vi "Build Coffee Shop.vi"(8 "error in (no error)":errorcluster) -> (0 "error out":errorcluster, 3 "Coffee Shop Out":refnum<class "Coffee Shop.lvclass">)   [LabVIEW 2020, in "Coffee Shop.lvclass"]
uses:
  Coffee Shop.lvclass
  Work Dispatcher/Work Dispatcher.lvclass
  C:/git/astemes-triarc-examples/source/Coffee Shop/Processes/People/Process Job/Job Handler.lvclass
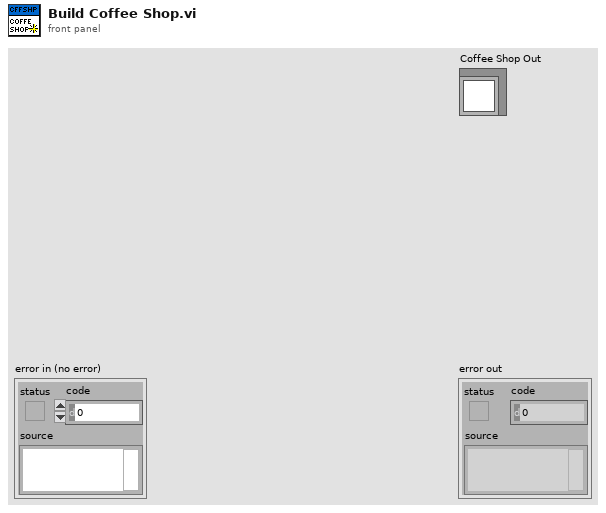
[diagram p1: front panel]
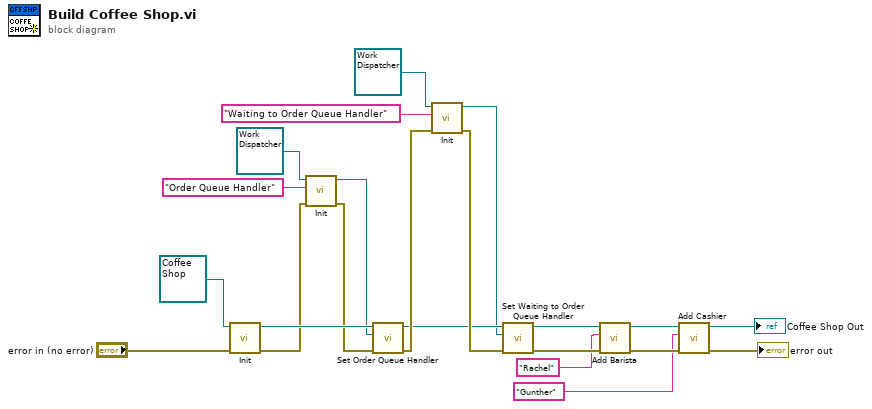
[diagram p0: block diagram]
diagram:
  n1 = call-dynamic "Init.vi"("error in (no error)"="error in (no error)", "Process In"=refnum<class "Coffee Shop.lvclass"> refnum ("Coffee Shop.lvclass")) -> ("error out"=w16:errorcluster, "Process Out"=w20:refnum<class "Coffee Shop.lvclass">)  [unwired: 8 in]
  n2 = call-dynamic "Init.vi"("error in (no error)"=w16, "Name"="Order Queue Handler", "Process In"=refnum<class "Work Dispatcher.lvclass"> refnum ("Work Dispatcher.lvclass")) -> ("error out"=w15:errorcluster, "Process Out"=w9:refnum<class "Work Dispatcher.lvclass">)  [unwired: 7 in]
  n3 = call "Set Order Queue Handler.vi"("error in (no error)"=w15, "Order Queue Handler"=w9, "Coffee Shop In"=w20) -> ("error out"=w13:errorcluster, "Coffee Shop Out"=w11:refnum<class "Coffee Shop.lvclass">)  [unwired: 7 in]
  n4 = call-dynamic "Init.vi"("error in (no error)"=w13, "Name"="Waiting to Order Queue Handler", "Process In"=refnum<class "Work Dispatcher.lvclass"> refnum ("Work Dispatcher.lvclass")) -> ("error out"=w12:errorcluster, "Process Out"=w10:refnum<class "Work Dispatcher.lvclass">)  [unwired: 7 in]
  n5 = call "Set Waiting to Order Queue Handler.vi"("error in (no error)"=w12, "Waiting To Order Queue Handler"=w10, "Coffee Shop In"=w11) -> ("error out"=w4:errorcluster, "Coffee Shop Out"=w3:refnum<class "Coffee Shop.lvclass">)  [unwired: 7 in]
  n6 = call "Add Barista.vi"("error in (no error)"=w4, "Name"="Rachel", "Coffee Shop in"=w3) -> ("error out"=w8:errorcluster, "Coffee Shop out"=w6:refnum<class "Coffee Shop.lvclass">)  [unwired: 7 in]
  n7 = call "Add Cashier.vi"("error in (no error)"=w8, "Name"="Gunther", "Coffee Shop in"=w6) -> ("error out"=→"error out":errorcluster, "Coffee Shop out"=→"Coffee Shop Out":refnum<class "Coffee Shop.lvclass">)  [unwired: 7 in]
